vi "Charact One Standard.vi"(0 "Vector Path in":refnum<class "Vector Path.lvclass">, 5 "Standard Type":T2, 11 "error in":errorcluster) -> (4 "Vector Path out":refnum<class "Vector Path.lvclass">, 6 "One-Port Charact Data":T1, 15 "error out":errorcluster)   [LabVIEW 2023, in "RFFixtureCharact.Public.lvlib" / "Vector Path.lvclass"]
uses:
  Vector Path.lvclass
  Instruments/Cal Standard/Type Definitions/Standard Type.ctl
  Instruments/Cal Standard/Type Definitions/One-Port Charact Data.ctl
  <vilib>/addons/_RFCalAndCharactDatabase/NI_RFCalAndCharact_Database_API.lvlibp/PXIe5633/Controls/Port Settings.ctl
  <vilib>/Utility/error.llb/Trim Whitespace.vi
  <vilib>/Utility/error.llb/Trim Whitespace One-Sided.vi
  <vilib>/RFmx/VNA/mx/RFmxVNA.llb/RFmxVNA Select Measurement (Single).vi
  <vilib>/RFmx/VNA/mx/RFmxVNA.llb/RFmxVNA SParams Fetch Complex Data.vi
  Instruments/Cal Standard/Cal Standard Base/Cal Standard Base.lvclass
  Instruments/Cal Standard/Cal Standard Factory/Cal Standard Factory.lvclass
  <resource>/objmgr/RFmxVNA.rc
  <vilib>/addons/_RFCalAndCharactDatabase/NI_RFCalAndCharact_Database_API.lvlibp/PXIe5633/PXIe5633.lvlib
  Instruments/RFFixtureCharact.Instruments.lvlib
  <resource>/objmgr/RFmxInstr.rc
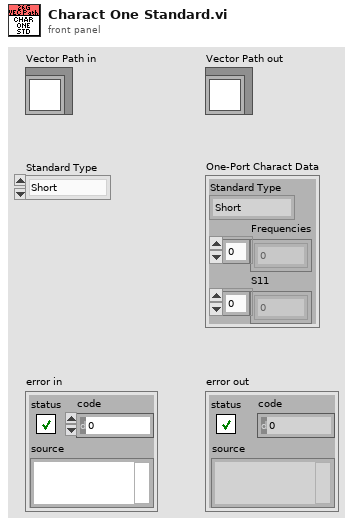
[diagram p1: front panel]
types:
  T1 = typedef "RFFixtureCharact.Instruments.lvlib/One-Port Charact Data.ctl" = cluster{"Standard Type":T2, "Frequencies":dbl[], "S11":cdb[]}
  T2 = typedef "RFFixtureCharact.Instruments.lvlib/Standard Type.ctl" = enum16{"Short", "Open", "Load", "PowerMeter", "None"}
  T3 = typedef "NI_RFCalAndCharact_Database_API.lvlibp/PXIe5633.lvlib/Port Settings.ctl" = cluster{"Port Name":string, "Power Level (dBm)":dbl, "Test Receiver Attenuation (dB)":dbl}
  T4 = typedef "RFFixtureCharact.Public.lvlib/Vector Path Group.lvclass/Sweep.ctl" = cluster{"Port Power":dbl, "Frequencies":dbl[], "Test Receiver Attenuation":dbl, "IF Bandwidth":dbl}
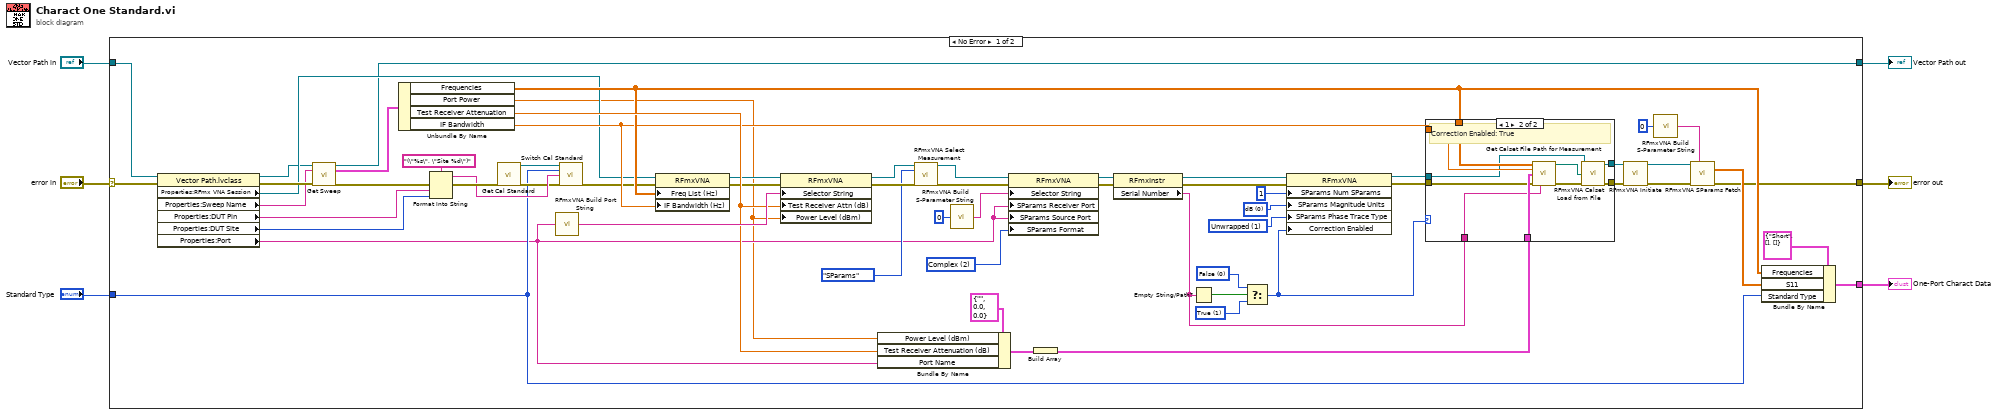
[diagram p0: block diagram]
diagram:
  n1 = case shown="No Error" "error in" {
    selector: "error in" -> [w66 w81]
    tunnel: [w12 w81] -> w5
    tunnel: [w9 w80] -> w3
    tunnel: "Vector Path in" -> [w67 w80]
    tunnel: "Standard Type" -> [w31 _]
    tunnel: [w13 _] -> w1
    frame No Error {
      w18 = 1 items=["False", "True"] ("Correction Enabled")
      w17 = 0 items=["False", "True"] ("Correction Enabled")
      w45 = 1 items=["Wrapped", "Unwrapped"] ("SParams Phase Trace Type")
      w46 = 0 items=["dB", "Linear"] ("SParams Magnitude Units")
      w50 = 2 items=["Magnitude", "Phase", "Complex"] ("SParams Format")
      n2 = property class="Vector Path.lvclass"(reference=w67, error in=w66) -> (reference out=w10:refnum<class "Vector Path.lvclass">, error out=w65:errorcluster, "Properties:RFmx VNA Session"=w14:refnum<k21>, "Properties:Sweep Name"=w11:string, "Properties:DUT Pin"=w58:string, "Properties:DUT Site"=w57:i32, "Properties:Port"=w30:string)
      n3 = call-dynamic "Get Sweep.vi"("Vector Path in"=w10, "Sweep Name"=w11, "error in (no error)"=w65) -> ("Vector Path out"=w9:refnum<class "Vector Path.lvclass">, "Sweep"=w8:T4, "error out"=w59:errorcluster)  [unwired: 9 in, 1 out]
      n4 = Unbundle By Name(w8) -> ("Frequencies"=w28:dbl[], "Port Power"=w7:dbl, "Test Receiver Attenuation"=w37:dbl, "IF Bandwidth"=w27:dbl)
      n5 = Format Into String(format string="(\"%s\", \"Site %d\")", error in=w59, w58, w57) -> (resulting string=w63:string, error out=w64:errorcluster)  [unwired: 1 in]
      n6 = call "Get Cal Standard.vi"("error in (no error)"=w64) -> ("Cal Standard Base out"=w61:refnum<class "Cal Standard Base.lvclass">, "error out"=w60:errorcluster)  [unwired: 12 in, 1 out]
      n7 = call <vilib>:"RFmxVNA Build Port String.vi"("Port Name"=w30) -> ("Selector String Out"=w56:string)  [unwired: 14 in]
      n8 = call-dynamic "Switch Cal Standard.vi"("Cal Standard Base in"=w61, "Standard Type"=w31, "Path Name"=w63, "error in (no error)"=w60) -> ("error out"=w15:errorcluster)  [unwired: 10 in, 1 out]
      n9 = property class="RFmxVNA"(reference=w14, error in=w15, "Freq List (Hz)"=w28, "IF Bandwidth (Hz)"=w27) -> (reference out=w34:refnum<k21>, error out=w33:errorcluster)
      n10 = property class="RFmxVNA"(reference=w34, error in=w33, "Selector String"=w56, "Test Receiver Attn (dB)"=w37, "Power Level (dBm)"=w7) -> (reference out=w54:refnum<k21>, error out=w55:errorcluster)
      n11 = Bundle By Name(cluster=T3 {"Port Name"="", "Power Level (dBm)"=0.0, "Test Receiver Attenuation (dB)"=0.0} ("Port Settings 2"), "Power Level (dBm)"=w7, "Test Receiver Attenuation (dB)"=w37, "Port Name"=w30) -> (w36:T3)
      n12 = call-poly <vilib>:"RFmxVNA Select Measurement.vi"("Instrument Handle In"=w54, "Measurement"=enum16{"SParams", "Waves"}."SParams", "error in (no error)"=w55) -> ("Instrument Handle Out"=w47:refnum<k21>, "error out"=w48:errorcluster)  [unwired: 11 in]
      n13 = call <vilib>:"RFmxVNA Build S-Parameter String.vi"("S-Parameter Number"=0) -> ("Selector String Out"=w51:string)  [unwired: 14 in]
      n14 = property class="RFmxVNA"(reference=w47, error in=w48, "Selector String"=w51, "SParams Receiver Port"=w30, "SParams Source Port"=w30, "SParams Format"=w50) -> (reference out=w24:refnum<k21>, error out=w23:errorcluster)
      n15 = Build Array(w36) -> (w35:T3[])
      n16 = property class="RFmxInstr"(reference=w24, error in=w23) -> (reference out=w22:refnum<k21>, error out=w21:errorcluster, "Serial Number"=w20:string)
      n17 = Empty String/Path?(string/path=w20) -> (empty?=w19:bool)
      n18 = Select(t=w17, s=w19, f=w18) -> (s? t:f=w16:i32)
      n19 = property class="RFmxVNA"(reference=w22, error in=w21, "SParams Num SParams"=1, "SParams Magnitude Units"=w46, "SParams Phase Trace Type"=w45, "Correction Enabled"=w16) -> (reference out=w25:refnum<k21>, error out=w26:errorcluster)
      n20 = case shown="1" w16 {
        tunnel: [w69 w79] -> w44
        tunnel: [w68 w78] -> w43
        tunnel: w35 -> [_ w77]
        tunnel: w28 -> [_ w74]
        tunnel: w27 -> [_ w73]
        tunnel: w26 -> [w69 w72]
        tunnel: w25 -> [w68 w71]
        tunnel: w20 -> [_ w70]
        frame 0, Default {
          # "Correction Enabled: False"
        }
        frame 1 {
          # "Correction Enabled: True"
          n21 = call <vilib>:"Get Calset File Path for Measurement.vi"("Frequency List (Hz)"=w74, "IF Bandwidth (Hz)"=w73, "Port Settings"=w77, "error in"=w72, "VNA Serial Number"=w70) -> ("Calset File Path"=w75:path, "error out"=w76:errorcluster)  [unwired: 8 in, 1 out]
          n22 = call <vilib>:"RFmxVNA Calset Load from File.vi"("Instrument Handle In"=w71, "Calset File Path"=w75, "error in (no error)"=w76) -> ("Instrument Handle Out"=w78:refnum<k21>, "error out"=w79:errorcluster)  [unwired: 11 in]
        }
      }
      n23 = call <vilib>:"RFmxVNA Initiate.vi"("Instrument Handle In"=w43, "error in (no error)"=w44) -> ("Instrument Handle Out"=w41:refnum<k21>, "error out"=w42:errorcluster)  [unwired: 11 in, 1 out]
      n24 = call <vilib>:"RFmxVNA Build S-Parameter String.vi"("S-Parameter Number"=0) -> ("Selector String Out"=w39:string)  [unwired: 14 in]
      n25 = call-poly <vilib>:"RFmxVNA SParams Fetch.vi"("Instrument Handle In"=w41, "Selector String"=w39, "error in (no error)"=w42) -> ("Complex Data"=w29:csg[], "error out"=w12:errorcluster)  [unwired: 10 in, 1 out]
      n26 = Bundle By Name(cluster=T1 {"Standard Type"=enum."Short", "Frequencies"=[], "S11"=[]} ("One-Port Charact Data"), "Frequencies"=w28, "S11"=w29, "Standard Type"=w31) -> (w13:T1)
    }
    frame Error {
    }
  }
  "error out" <- w5
  "Vector Path out" <- w3
  "One-Port Charact Data" <- w1
